vi "execute.vi"(8 "error in (no error)":errorcluster, 10 "Context in":refnum<class "Context.lvclass">, 11 "StandbyCommand in":refnum<class "StandbyCommand.lvclass">) -> (0 "error out":errorcluster, 2 "Context out":refnum<class "Context.lvclass">, 3 "StandbyCommand out":refnum<class "StandbyCommand.lvclass">)   [LabVIEW 2016, in "StandbyCommand.lvclass"]
uses:
  StandbyCommand.lvclass
  Context/Context.lvclass
  StandbyCommand.lvclass/StandbyCommand.ctl
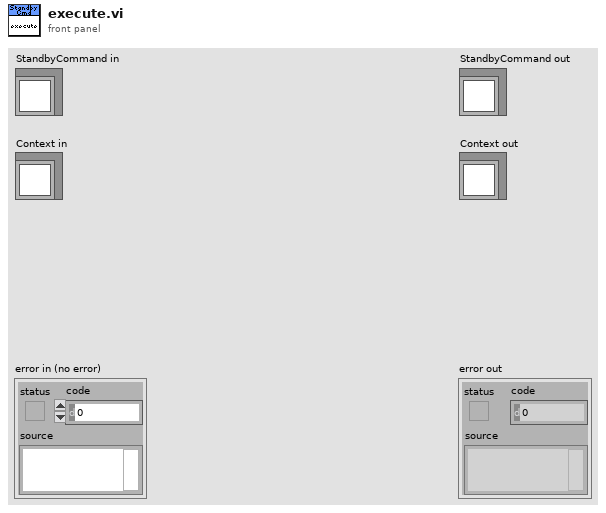
[diagram p1: front panel]
types:
  T1 = typedef "M1M3SupportTopics.lvlib/CommandStandby.ctl" = cluster{"CommandId":T2, "Standby":bool}
  T2 = typedef "M1M3SupportTopics.lvlib/CommandId.ctl" = i32
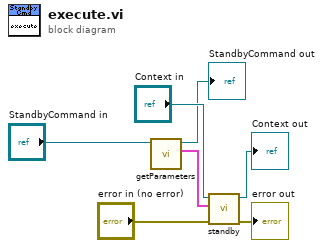
[diagram p0: block diagram]
diagram:
  n1 = call "getParameters.vi"("StandbyCommand in"="StandbyCommand in") -> ("Parameters"=w3:T1, "StandbyCommand out"=→"StandbyCommand out":refnum<class "StandbyCommand.lvclass">)  [unwired: 9 in]
  n2 = call-dynamic "standby.vi"("error in (no error)"="error in (no error)", "Parameters"=w3, "Context in"="Context in") -> ("error out"=→"error out":errorcluster, "Context out"=→"Context out":refnum<class "Context.lvclass">)  [unwired: 7 in]
